vi "Measure Ru.vi"(8 "Arduino In":T8, 10 "reference in":refnum<vi>, 11 "Ring in":refnum<vi>) -> (0 "Arduino Out":T7, 1 "f":dbl, 3 "Ru":dbl, 5 "Vo":dbl)   [LabVIEW 2022 SP3]
uses:
  <vilib>/MakerHub/LINX/Private/Type Defs/LINX Ref.ctl
  <vilib>/MakerHub/LINX/Private/Type Defs/Platform.ctl
  <vilib>/MakerHub/LINX/Private/Type Defs/Interface.ctl
  <vilib>/MakerHub/LINX/Private/Device/Type Defs/LINX Device Config.ctl
  <vilib>/MakerHub/LINX/Private/Device/Type Defs/TCP Config.ctl
  <vilib>/MakerHub/LINX/Private/Device/Type Defs/Channels.ctl
  <vilib>/MakerHub/LINX/Public/Peripherals/PWM/PWM Set Duty Cycle 1 Chan.vi
  <vilib>/MakerHub/LINX/Public/Peripherals/Analog/Analog Read 1 Chan.vi
  <vilib>/MakerHub/LINX/Public/Peripherals/Analog/Analog Read N Chans.vi
  <vilib>/MakerHub/LINX/Private/Local IO/LinxAnalogRead.vi
  <vilib>/MakerHub/LINX/Public/Utilities/Check Channel.vi
  <vilib>/MakerHub/LINX/Public/Peripherals/PWM/PWM Set Duty Cycle N Chans.vi
  <vilib>/MakerHub/LINX/Private/Utilties/Generate Error.vi
  <vilib>/MakerHub/LINX/LMH-LINX.lvlib
  <vilib>/MakerHub/LINX/Private/Device/Device.lvlib
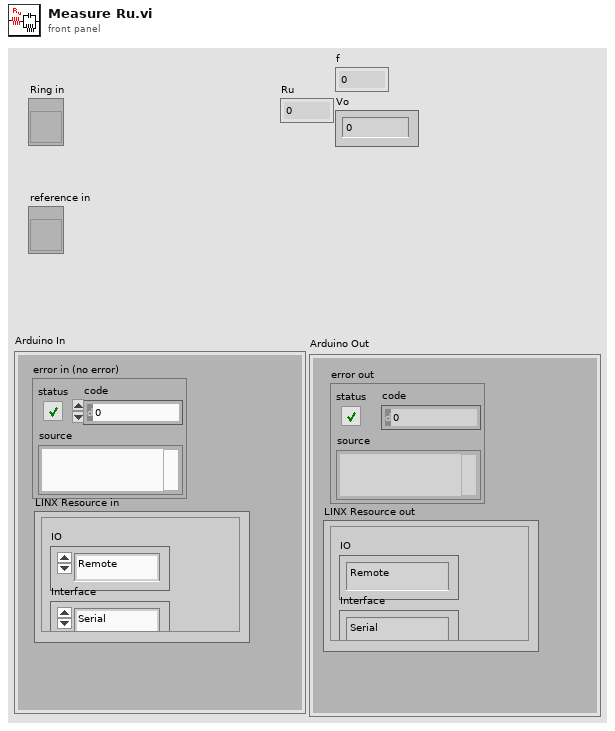
[diagram p1: front panel]
types:
  T1 = typedef "LMH-LINX.lvlib/LINX Ref.ctl" = cluster{"IO":T2, "Interface":T3, "LINX Device Config":T4}
  T2 = typedef "LMH-LINX.lvlib/Platform.ctl" = enum16{"Remote", "Local"}
  T3 = typedef "LMH-LINX.lvlib/Interface.ctl" = enum16{"Serial", "TCP"}
  T4 = typedef "LMH-LINX.lvlib/Device.lvlib/LINX Device Config.ctl" = cluster{"Interface":T3, "COM Port":refnum<visa-resource-name>, "TCP Configuration":T5, "Device Family":u8, "Device ID":u8, "Device Name":string, "TCP Ref":refnum<k5>, "Channels":T6}
  T5 = typedef "LMH-LINX.lvlib/Device.lvlib/TCP Config.ctl" = cluster{"IP Address":string, "Port":u16}
  T6 = typedef "LMH-LINX.lvlib/Channels.ctl" = cluster{"DI":u8[], "DO":u8[], "AI":u8[], "AO":u8[], "PWM":u8[], "QE":u8[], "UART":u8[], "I2C 2":u8[], "SPI":u8[], "CAN":u8[], "Servo":u8[], "AI Ref (V)":dbl, "AI Resolution (Bits)":u8, "AO Ref (V)":dbl, "AO Resolution (Bits)":u8}
  T7 = cluster{"error out":errorcluster, "LINX Resource out":T1}
  T8 = cluster{"error in (no error)":errorcluster, "LINX Resource in":T1}
  T9 = cluster{"Error Out":errorcluster, "LINX Resource":T1}
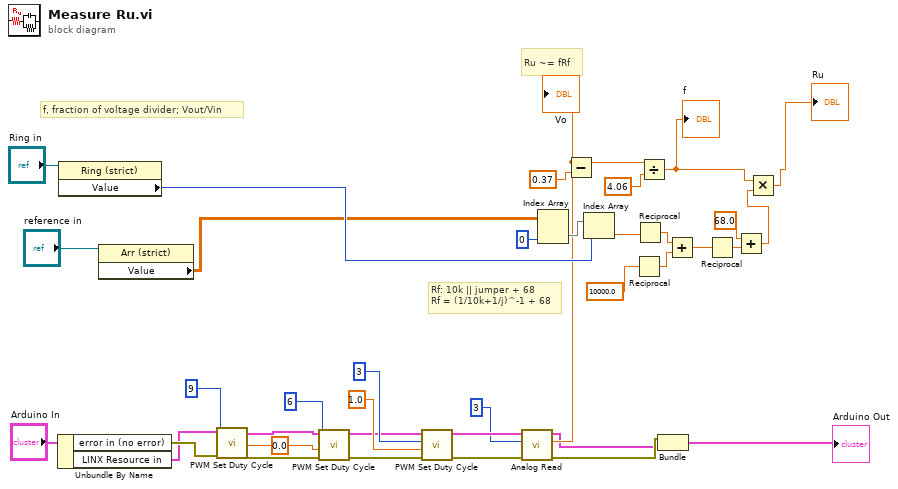
[diagram p0: block diagram]
diagram:
  w9 = 0.0 ("Duty Cycle (0-1)")
  # "Ru ~= fRf"
  # "f, fraction of voltage divider; Vout/Vin"
  # "Rf: 10k || jumper + 68\nRf = (1/10k+1/j)^-1 + 68"
  n1 = Unbundle By Name("Arduino In") -> ("error in (no error)"=w5:errorcluster, "LINX Resource in"=w4:T1)
  n2 = property class="Ring (strict)"(reference="Ring in") -> ("Value"=w28:u16)  [unwired: 1 in, 2 out]
  n3 = property class="Arr (strict)"(reference="reference in") -> ("Value"=w25:dbl[][])  [unwired: 1 in, 2 out]
  n4 = call-poly <vilib>:"PWM Set Duty Cycle.vi"("Error In"=w5, "Duty Cycle (0-1)"=w9, "PWM Channel"=u8 9, "LINX Resource"=w4) -> ("Error Out"=w11:errorcluster, "LINX Resource"=w12:T1)  [unwired: 6 in]
  n5 = call-poly <vilib>:"PWM Set Duty Cycle.vi"("Error In"=w11, "Duty Cycle (0-1)"=w9, "PWM Channel"=u8 6, "LINX Resource"=w12) -> ("Error Out"=w10:errorcluster, "LINX Resource"=w13:T1)  [unwired: 6 in]
  n6 = call-poly <vilib>:"PWM Set Duty Cycle.vi"("Error In"=w10, "Duty Cycle (0-1)"=1.0, "PWM Channel"=u8 3, "LINX Resource"=w13) -> ("Error Out"=w21:errorcluster, "LINX Resource"=w20:T1)  [unwired: 6 in]
  n7 = call-poly <vilib>:"Analog Read.vi"("Error In"=w21, "Analog Channel"=u8 3, "LINX Resource"=w20) -> ("Error Out"=w3:errorcluster, "Voltage"=w23:dbl, "LINX Resource"=w2:T1)  [unwired: 5 in, 1 out]
  "Vo" <- w23
  n8 = Index Array(array=w25, index (col)=0 ("disabled index (col)")) -> (element=w27:dbl[])  [unwired: 1 in]
  n9 = Subtract(x=w23, y=0.37) -> (x-y=w15:dbl)
  n10 = Index Array(array=w27, index=w28) -> (element=w29:dbl)
  n11 = Reciprocal(x=10000.0) -> (1/x=w32:dbl)
  n12 = Reciprocal(x=w29) -> (1/x=w31:dbl)
  n13 = Divide(x=w15, y=4.06) -> (x/y=w38:dbl)
  "f" <- w38
  n14 = Bundle("Error Out"=w3, "LINX Resource"=w2) -> (→"Arduino Out":T9)  [unwired: 1 in]
  n15 = Add(x=w31, y=w32) -> (x+y=w33:dbl)
  n16 = Reciprocal(x=w33) -> (1/x=w34:dbl)
  n17 = Add(x=68.0, y=w34) -> (x+y=w36:dbl)
  n18 = Multiply(x=w38, y=w36) -> (x*y=→"Ru":dbl)
